vi "test 3-icon-demo.vi"() -> ()   [LabVIEW 2019]
uses:
  _ctrl/BP4610_config.ctl
  _ctrl/BP4610_return.ctl
  _ctrl/rw.ctl
panel:
  out "output 2":T1 {"DC current[A]" format="%.2f"; "DC voltage[V]" format="%.1f"}
  out "error out":errorcluster
  in  "BP4610 Config":T2={"VISA"="USB0::0x0D4A::0x0040::9426269::INSTR", "Limit-BP"={"Set"=enum."Current", "Voltage+[V]"=20.0, "Current+[A]"=5.0, "Voltage-[V]"=-20.0, "Current-[A]"=-5.0}, "SET BP"={"Set"=enum."FREQ/WAVE", "Operation mode"=0, "Voltage[Vp-p]"=10.0, "Current[Ap-p]"=2.0, "Voltage[V]"=-10.0, "Current[A]"=1.0, "Frequency[Hz]"=1.0, "Waveform"=enum."Sine"}, "Output"=FALSE} {"SET BP"."Frequency[Hz]" min=1.0 max=100000.0 step=0.1; "SET BP"."Current[A]" min=-20.0 max=20.0 step=0.001; "SET BP"."Voltage[V]" min=-20.0 max=20.0 step=0.001; "SET BP"."Current[Ap-p]" min=-115.0 max=115.0 step=0.01; "SET BP"."Voltage[Vp-p]" min=0.0 max=60.0 step=0.01; "SET BP"."Operation mode" items=["CV-INT", "CV-EXT", "CV-ADD", "CC-INT", "CC-EXT", "CC-ADD"]; "Limit-BP"."Current-[A]" min=-20.0 max=20.0 step=0.001; "Limit-BP"."Voltage-[V]" min=-115.0 max=115.0 step=0.01; "Limit-BP"."Current+[A]" min=0.0 max=60.0 step=0.01; "Limit-BP"."Voltage+[V]" min=0.0 max=120.0 step=0.1}
  in  "cmd":enum16{"limit", "output", "set", "read"}(ring)=enum."set"
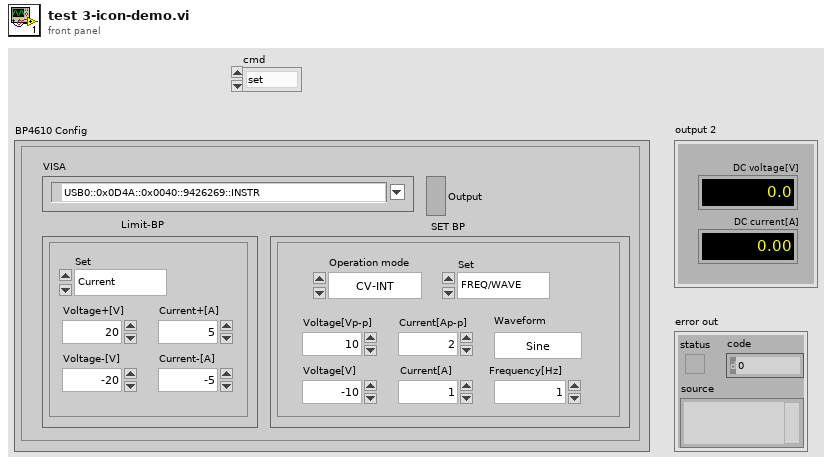
[diagram p1: front panel]
types:
  T1 = typedef "BP4610_return.ctl" = cluster{"DC voltage[V]":dbl, "DC current[A]":dbl}
  T2 = typedef "BP4610_config.ctl" = cluster{"VISA":refnum<visa-resource-name>, "Limit-BP":cluster{"Set":enum16{"Current", "Voltage"}, "Voltage+[V]":dbl, "Current+[A]":dbl, "Voltage-[V]":dbl, "Current-[A]":dbl}, "SET BP":cluster{"Set":enum16{"Current", "Voltage", "FREQ/WAVE"}, "Operation mode":u16, "Voltage[Vp-p]":dbl, "Current[Ap-p]":dbl, "Voltage[V]":dbl, "Current[A]":dbl, "Frequency[Hz]":dbl, "Waveform":enum16{"Sine", "Square", "ARB 1", "ARB 2", "ARB 3", "ARB 4", "ARB 5", "ARB 6", "ARB 7", "ARB 8", "ARB 9", "ARB 10", "ARB 11", "ARB 12", "ARB 13", "ARB 14", "ARB 15", "ARB 16"}}, "Output":bool}
  T3 = typedef "rw.ctl" = enum16{"read", "write"}
  T4 = cluster{"Set":enum16{"Current", "Voltage"}, "Voltage+[V]":dbl, "Current+[A]":dbl, "Voltage-[V]":dbl, "Current-[A]":dbl}
  T5 = cluster{"Set":enum16{"Current", "Voltage", "FREQ/WAVE"}, "Operation mode":u16, "Voltage[Vp-p]":dbl, "Current[Ap-p]":dbl, "Voltage[V]":dbl, "Current[A]":dbl, "Frequency[Hz]":dbl, "Waveform":enum16{"Sine", "Square", "ARB 1", "ARB 2", "ARB 3", "ARB 4", "ARB 5", "ARB 6", "ARB 7", "ARB 8", "ARB 9", "ARB 10", "ARB 11", "ARB 12", "ARB 13", "ARB 14", "ARB 15", "ARB 16"}}
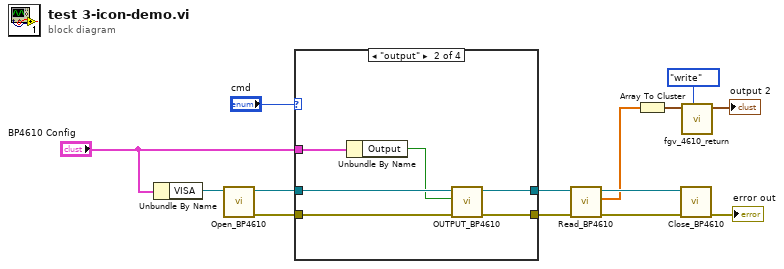
[diagram p0: block diagram]
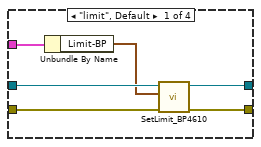
[diagram p2: hidden frame]
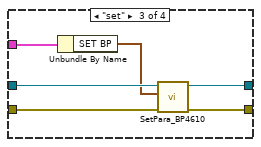
[diagram p3: hidden frame]
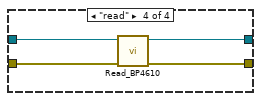
[diagram p4: hidden frame]
diagram:
  n1 = Unbundle By Name("BP4610 Config") -> ("VISA"=w1:refnum<visa-resource-name>)
  n2 = call "Open_BP4610.vi"("VISAsession"=w1) -> ("error out"=w13:errorcluster, "CopyVISAsession"=w14:refnum<visa-resource-name>)  [unwired: 9 in]
  n3 = case shown="\"output\"" "cmd" {
    tunnel: w14 -> [w20 w25 w29 w36]
    tunnel: w13 -> [w19 w26 w30 w34]
    tunnel: [w18 w24 w31 w33] -> w10
    tunnel: [w17 w23 w32 w35] -> w7
    tunnel: "BP4610 Config" -> [w16 w22 w28 _]
    frame "limit", Default {
      n4 = Unbundle By Name(w16) -> ("Limit-BP"=w15:T4)
      n5 = call "SetLimit_BP4610.vi"("error in"=w19, "LimitBP"=w15, "VISA"=w20) -> ("error out"=w18:errorcluster, "VISA out"=w17:refnum<visa-resource-name>)  [unwired: 7 in]
    }
    frame "output" {
      n6 = Unbundle By Name(w22) -> ("Output"=w21:bool)
      n7 = call "OUTPUT_BP4610.vi"("error in"=w26, "Output"=w21, "port in"=w25) -> ("error out"=w24:errorcluster, "port out"=w23:refnum<visa-resource-name>)  [unwired: 7 in]
    }
    frame "set" {
      n8 = Unbundle By Name(w28) -> ("SET BP"=w27:T5)
      n9 = call "SetPara_BP4610.vi"("error in"=w30, "SetBP"=w27, "VISA"=w29) -> ("error out"=w31:errorcluster, "VISA out"=w32:refnum<visa-resource-name>)  [unwired: 7 in]
    }
    frame "read" {
      n10 = call "Read_BP4610.vi"("error in (no error)"=w34, "VISAsession"=w36) -> ("error out"=w33:errorcluster, "CopyVISAsession"=w35:refnum<visa-resource-name>)  [unwired: 7 in, 1 out]
    }
  }
  n11 = call "Read_BP4610.vi"("error in (no error)"=w10, "VISAsession"=w7) -> ("error out"=w9:errorcluster, "Data"=w4:dbl[], "CopyVISAsession"=w8:refnum<visa-resource-name>)  [unwired: 7 in]
  n12 = Array To Cluster(array=w4) -> (cluster=w3:cluster{"Data[0]":dbl, "Data[1]":dbl})
  n13 = call "Close_BP4610.vi"("error in"=w9, "VISA"=w8) -> ("error out"=→"error out":errorcluster)  [unwired: 9 in]
  n14 = call "fgv_4610_return.vi"("cmd"=rw."write", "output"=w3) -> ("output 2"=→"output 2":T1)  [unwired: 9 in]
